vi "Waveform and Laser Controls V4.vi"() -> ()   [LabVIEW 2014]
uses:
  Waveform Scan Parameters.ctl
  <vilib>/Platform/TimedLoop/XDataNode/timing_clust.ctl
  <vilib>/Platform/TimedLoop/XDataNode/nitl_modes.ctl
  <vilib>/Platform/TimedLoop/XDataNode/wakeup.ctl
  <vilib>/rvi/Emulation/niFpgaGetClockAttributes.vi
  <vilib>/rvi/Emulation/niFpgaSctlEmulationGetInTimedLoop.vi
  <vilib>/rvi/Emulation/niFpgaEmulationReportErrorSimple.vi
  <vilib>/rvi/Emulation/niFpgaProcessEmulError.vi
  <vilib>/rvi/eio/common/nirviEmuTemplateMethod_errors.vi
  <vilib>/rvi/Emulation/niFpgaCriticalErrorInLSC.vi
  <vilib>/rvi/Memory/Memory_Emulation/nirvimemoryFastEmulation.vi
  <vilib>/rvi/Memory/Memory_Emulation/nirvimemoryEmulation.vi
  <vilib>/rvi/Emulation/niFpgaEmulationIsFPGAContextNoSignature.vi
  <vilib>/rvi/DataTransferAndStorage/Container/Common/niFpgaContainerGetUniqueNameForEmu.vi
  <vilib>/rvi/errors/nirviReportUnexpectedCaseInternalError (U32).vi
  <vilib>/eio/EIONode/EIONode.xnode
  <vilib>/rvi/DataTransferAndStorage/Container/XNode/niFpgaContainer.xnode
  <vilib>/Platform/TimedLoop/XDataNode/XDataNode.xnode
  <vilib>/Platform/TimedLoop/XDataNode/XDNodeRunTimeDep.lvlib
panel:
  in  "775 AOM (I16)":i16=16500
  in  "590 Analog Voltage (I16)":i16
  out "Laser Blank Trigger":bool
  in  "Laser On Time (Ticks)":u8=8
  in  "Sequences":u8=4
  in  "Laser Delay (Ticks)":u8
  in  "Laser States":u32
  in  "Blanking Off/Manual":bool
  in  "Z Piezo Axis":i16
  in  "Y Piezo Axis":i16
  in  "X Piezo Axis":i16
  out "End Linear Ramp":bool
  in  "End of Linear Ramp":u32
  in  "Z Stack Start Position (I16)":i16
  in  "Frames Per Z Step":u8
  in  "Number of Z Steps":u8
  in  "Z Step Size (I16)":i16
  in  "Stop Sync Signal":bool
  in  "Accums Per Line":u32[](array[numeric])=[0, 0, 0, 0]
  in  "Number of Lines":u32
  out "Frame Trigger":bool
  in  "Reset Position Error":bool
  in  "Galvo 1 Position (I16)":i16
  in  "Galvo 2 Position (I16)":i16
  in  "WF 3 Data Loaded":bool
  in  "WF 2 Data Loaded":bool
  in  "Waveform Scan Parameters":T1={"Scanning Mode"=0, "Fast Axis WF Length (Elements)"=0, "Fast Axis Sample Period (Ticks)"=40, "Slow Axis 1 WF Length (Elements)"=0, "Slow Axis 1 Sample Period (Ticks)"=40, "Slow Axis 1 Delay (25 ns) Steps"=40, "Slow Axis 2 WFLength (Elements)"=0, "Slow Axis 2 Sample Period (Ticks)"=40, "Slow Axis 2 Delay (25 ns) Steps"=40}
  in  "Resonant Mirror":T2
  in  "Galvo Mirror 2":T3
  in  "Galvo Mirror 1":T3
  in  "Start Waveforms":bool
  in  "Unused Axis Offset":i16
  in  "Slow Axis 2 Waveform Element":i16
  in  "Fast Axis Waveform Element":i16
  in  "Slow Axis 1 Waveform Element":i16
  in  "WF 1 Data Loaded":bool
  # "V2 - Adding in a line clock\nV3 - Cluster Scan Parameters"
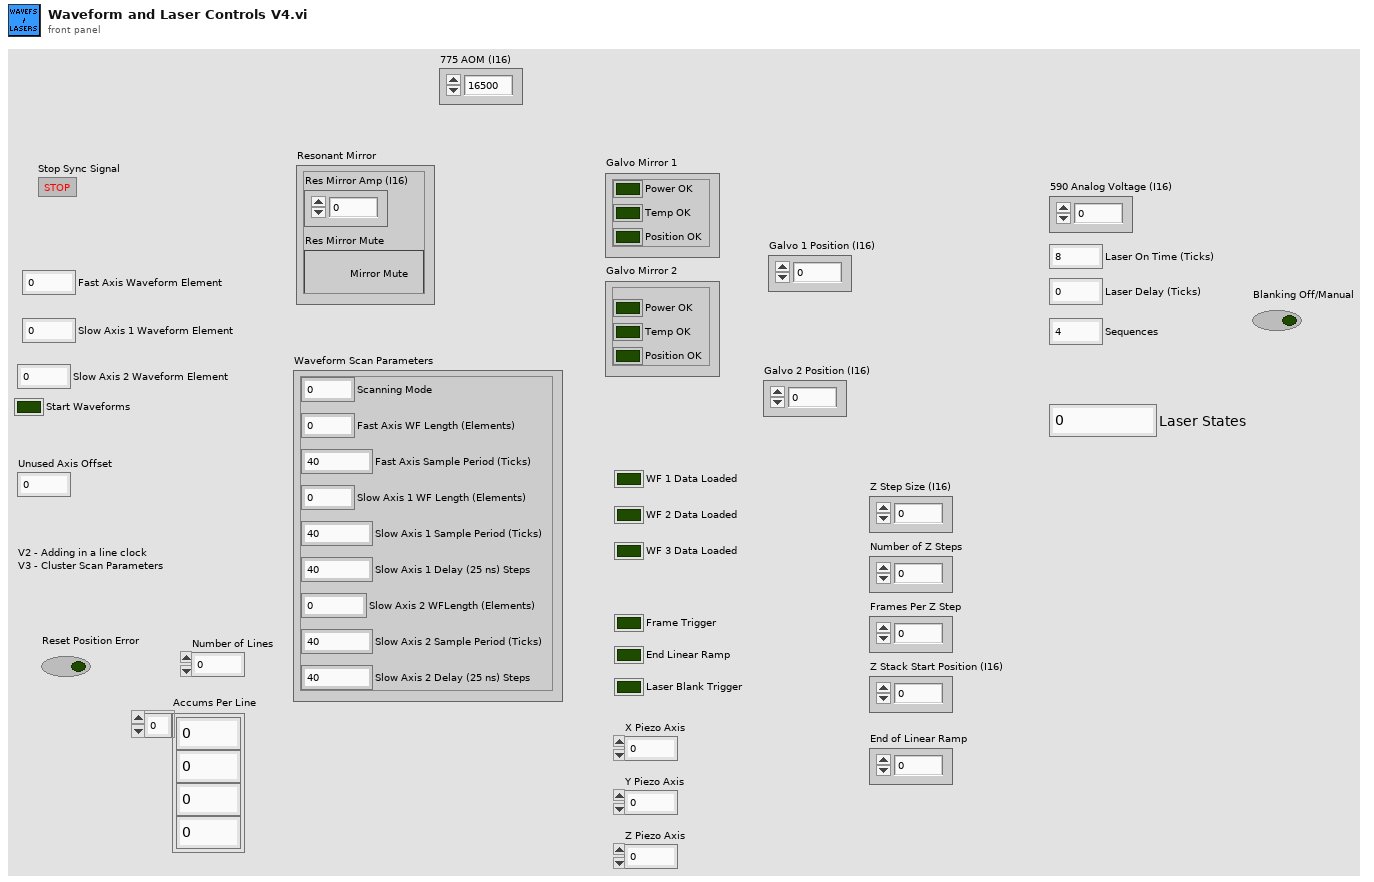
[diagram p1: front panel]
types:
  T1 = typedef "Waveform Scan Parameters.ctl" = cluster{"Scanning Mode":u8, "Fast Axis WF Length (Elements)":i32, "Fast Axis Sample Period (Ticks)":u32, "Slow Axis 1 WF Length (Elements)":i32, "Slow Axis 1 Sample Period (Ticks)":u32, "Slow Axis 1 Delay (25 ns) Steps":i32, "Slow Axis 2 WFLength (Elements)":i32, "Slow Axis 2 Sample Period (Ticks)":u32, "Slow Axis 2 Delay (25 ns) Steps":i32}
  T2 = cluster{"Res Mirror Amp (I16)":i16, "Res Mirror Mute":bool}
  T3 = cluster{"Power OK":bool, "Temp OK":bool, "Position OK":bool}
  T4 = typedef "XDNodeRunTimeDep.lvlib/timing_clust.ctl" = cluster{"Expected End [f-1]":u64, "Actual End [f-1]":u64, "Finished Late? [f-1]":bool, "Expected End [i-1]":u64, "Actual End [i-1]":u64, "Finished Late? [i-1]":bool, "Expected Start [i]":u64, "Actual Start [i]":u64, "Expected Start [f]":u64, "Actual Start [f]":u64, "Source Name":string, "Structure Name":string, "Period":i64, "Deadline":i64, "Offset":i64, "Start":i64, "Priority":i32, "Timeout":i32, "Mode":T5, "Wakeup Reason":T6, "Error":errorcluster, "Source Type":string, "Secondary Source Type":string, "Global End Time":u64, "Global Start Time":u64, "Frame Duration":u64, "Iteration Duration":u64, "Assigned CPU":i32, "I/O Scan Engine Mode":u32}
  T5 = typedef "XDNodeRunTimeDep.lvlib/nitl_modes.ctl" = enum32{"No Change", "Process missed periods, maintain original phase", "Discard missed periods, maintain original phase", "Process missed periods, ignore original phase", "Discard missed periods, ignore original phase"}
  T6 = typedef "XDNodeRunTimeDep.lvlib/wakeup.ctl" = enum32{"Normal", "Aborted", "Asynchronous wakeup", "Timing source error", "Timed loop error", "Timeout"}
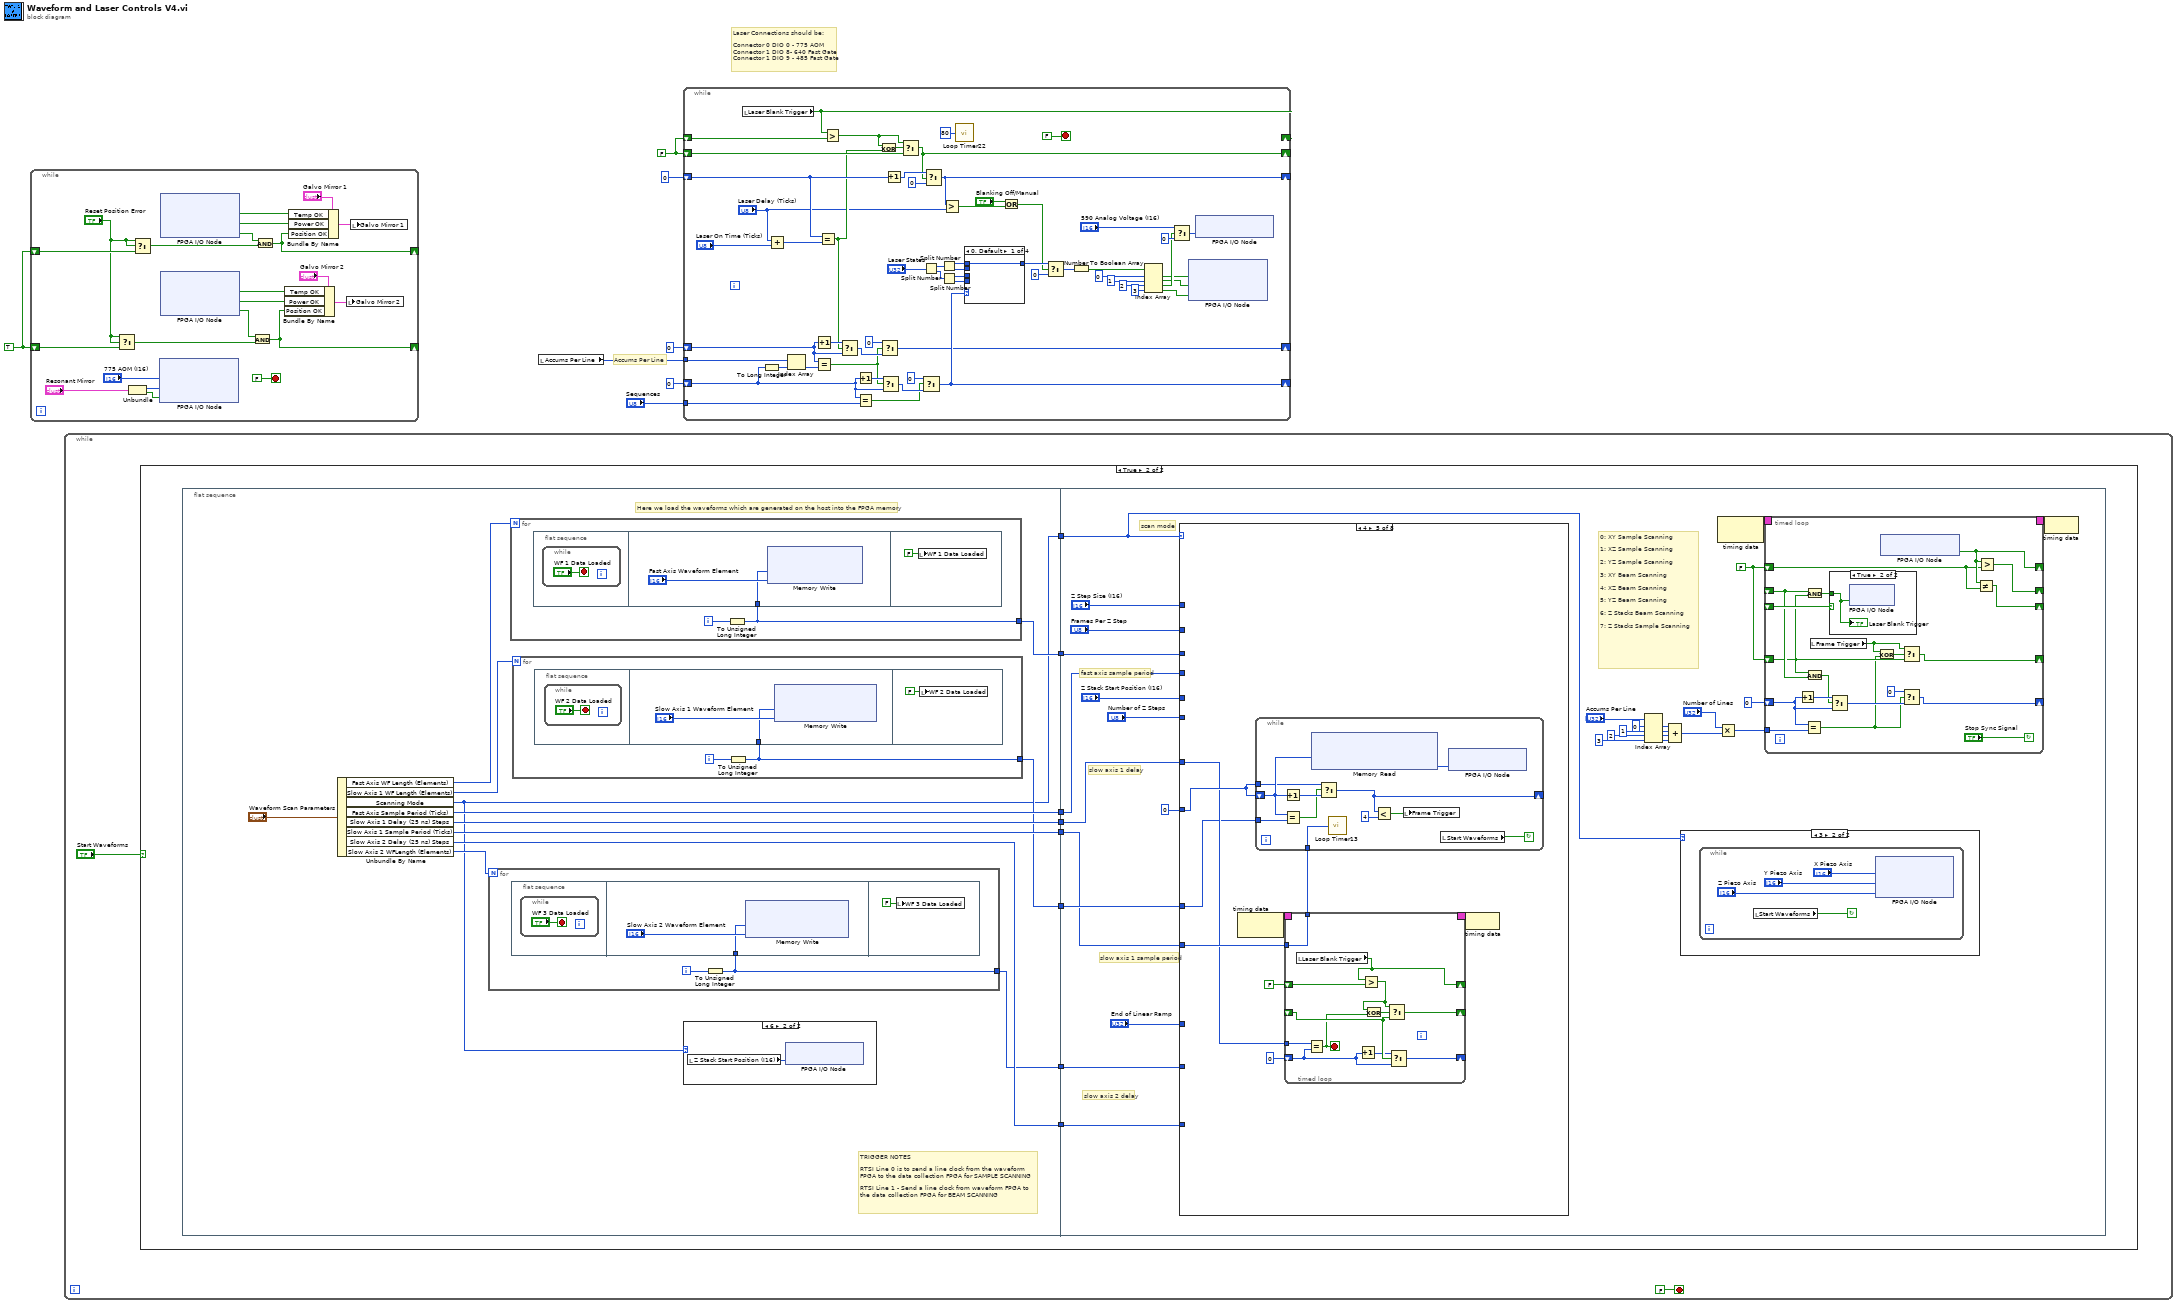
[diagram p0: block diagram]
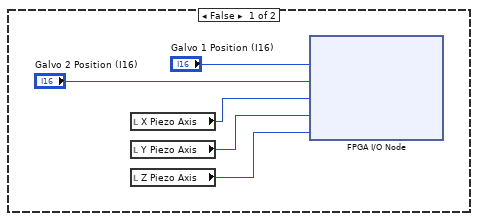
[diagram p5: hidden frame]
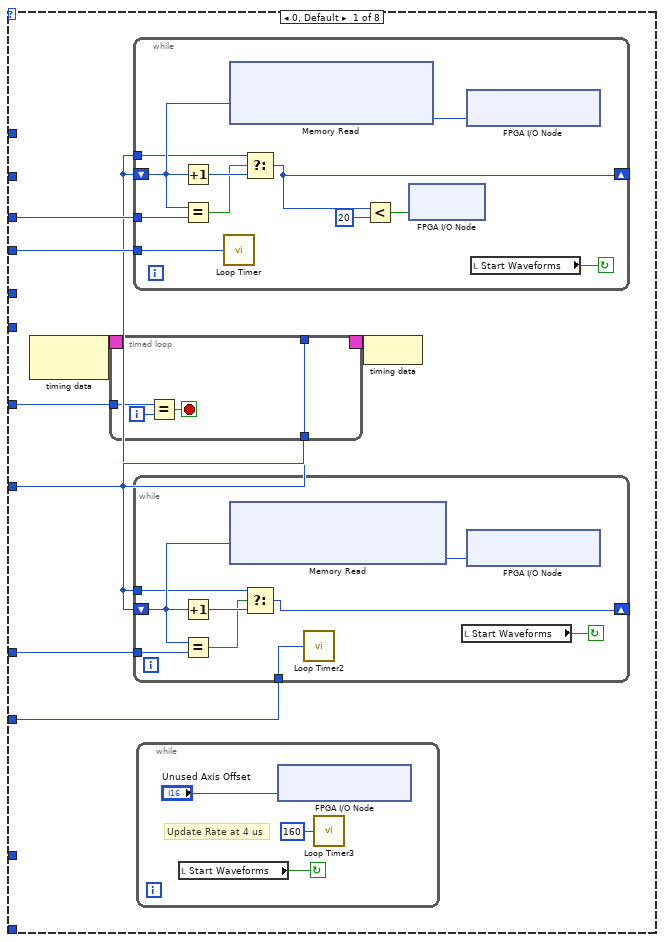
[diagram p9: hidden frame]
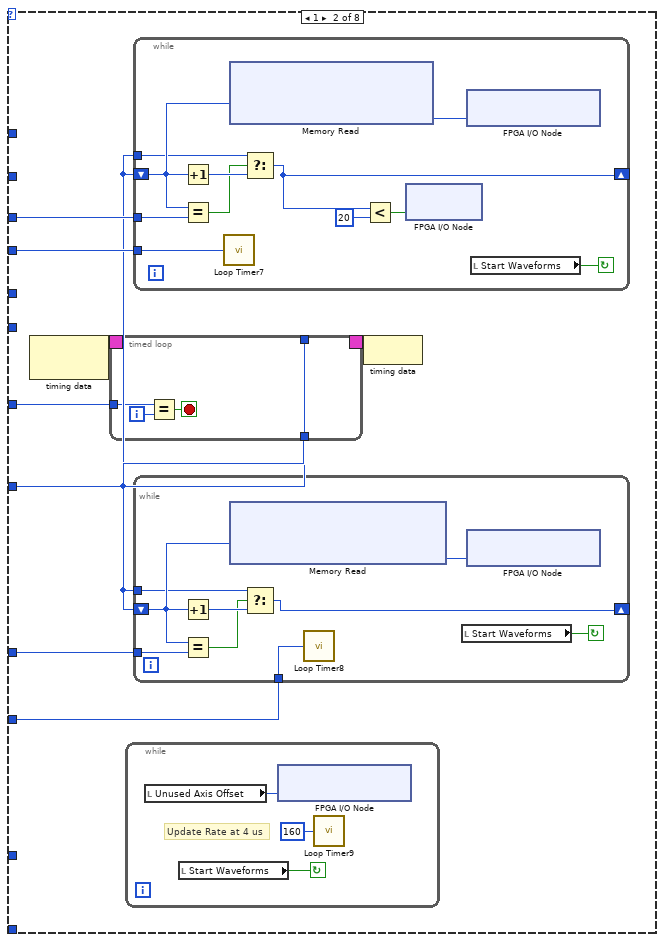
[diagram p10: hidden frame]
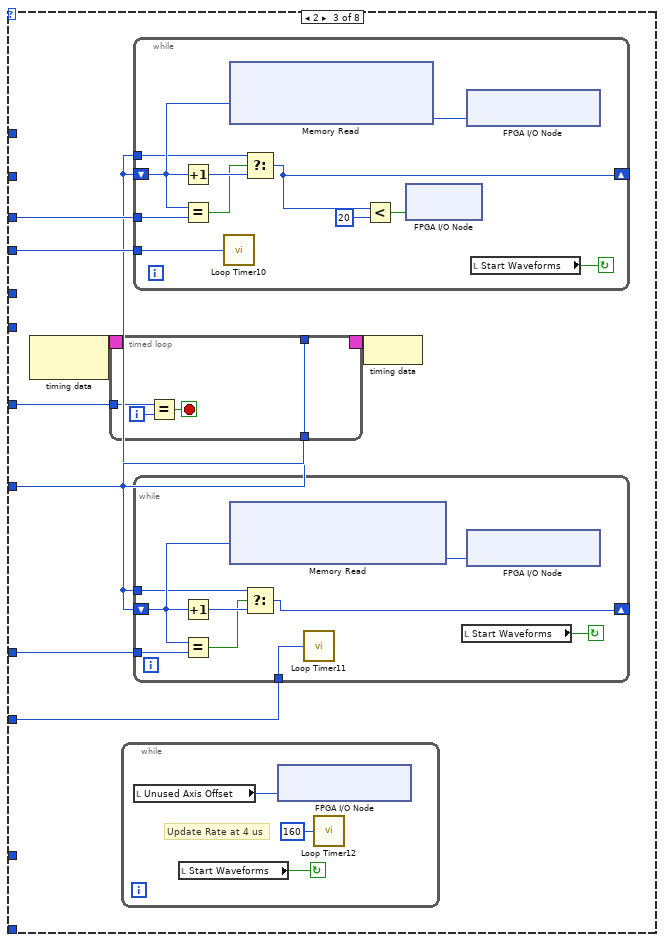
[diagram p11: hidden frame]
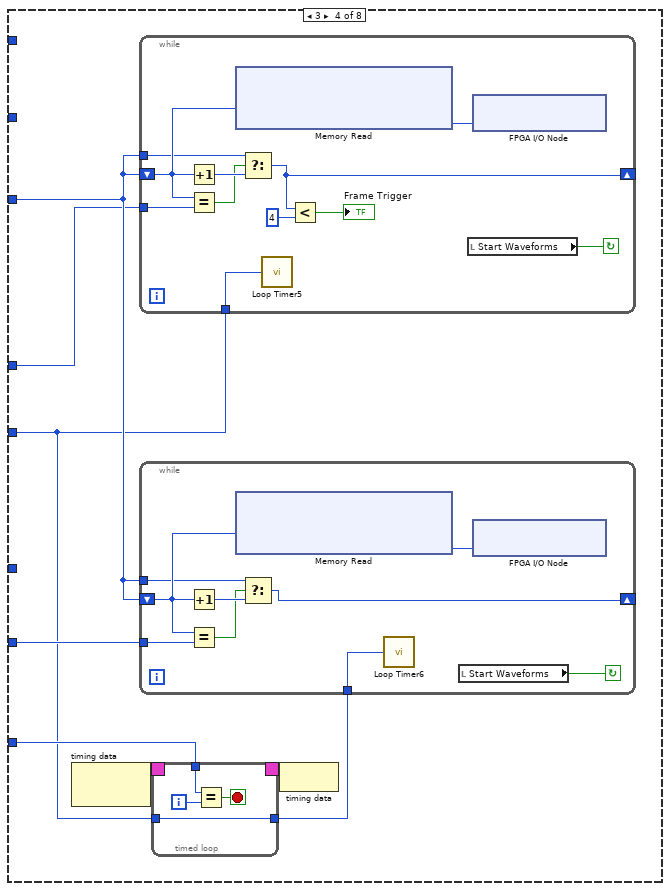
[diagram p12: hidden frame]
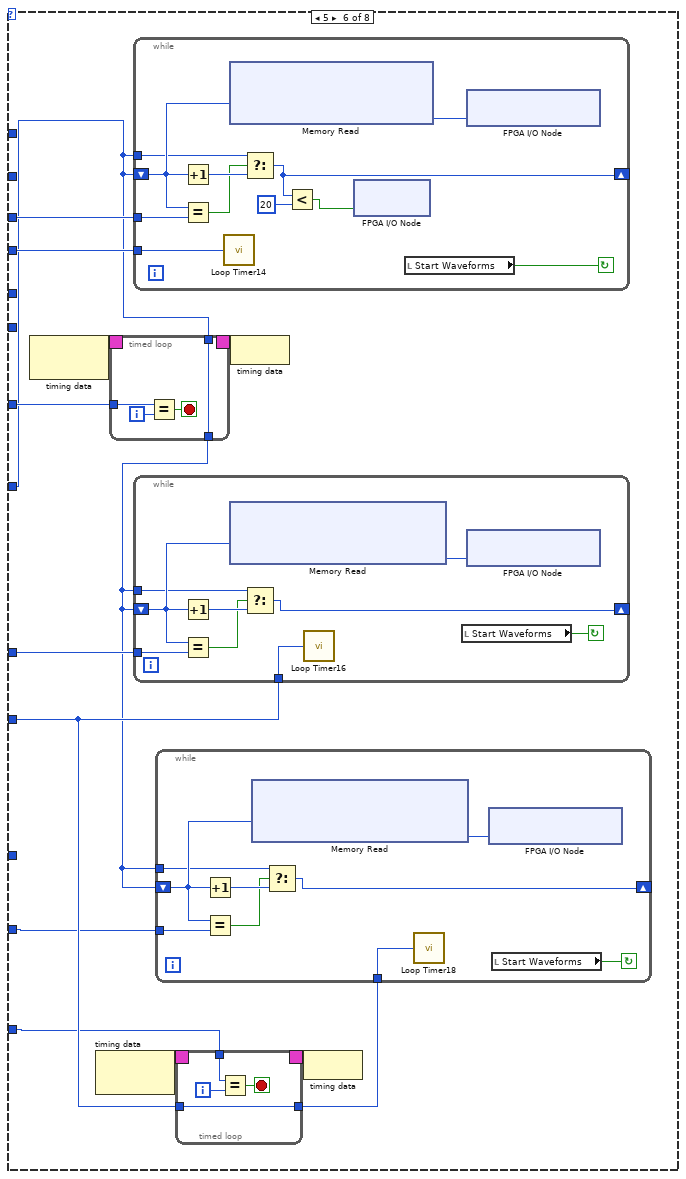
[diagram p13: hidden frame]
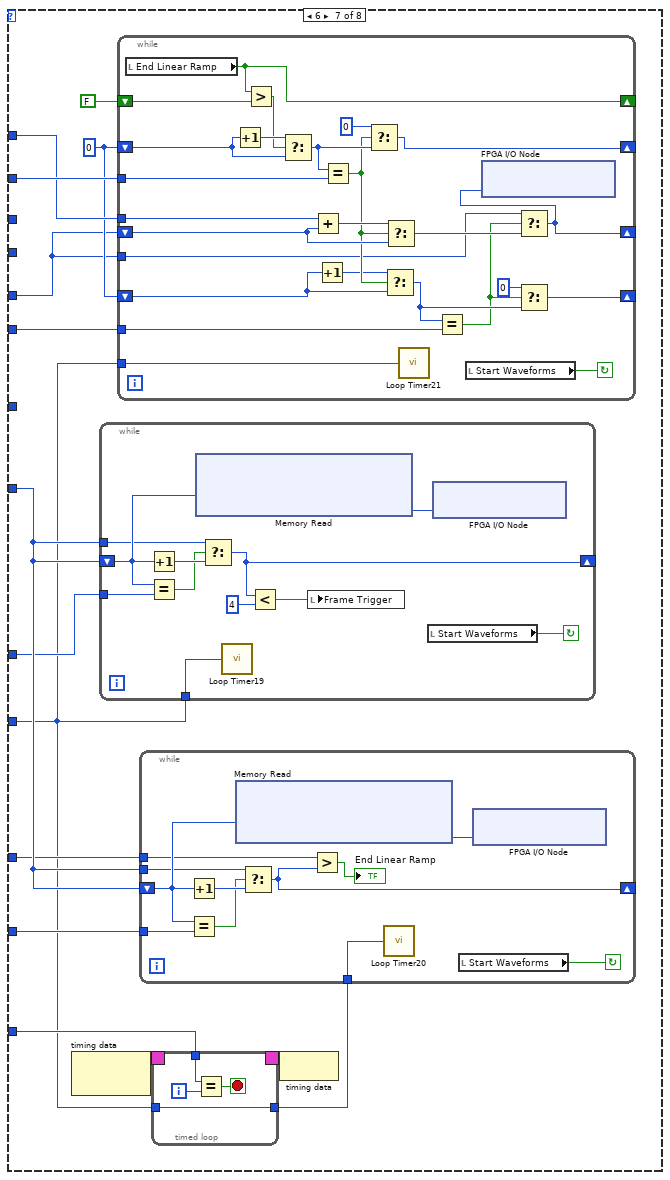
[diagram p14: hidden frame]
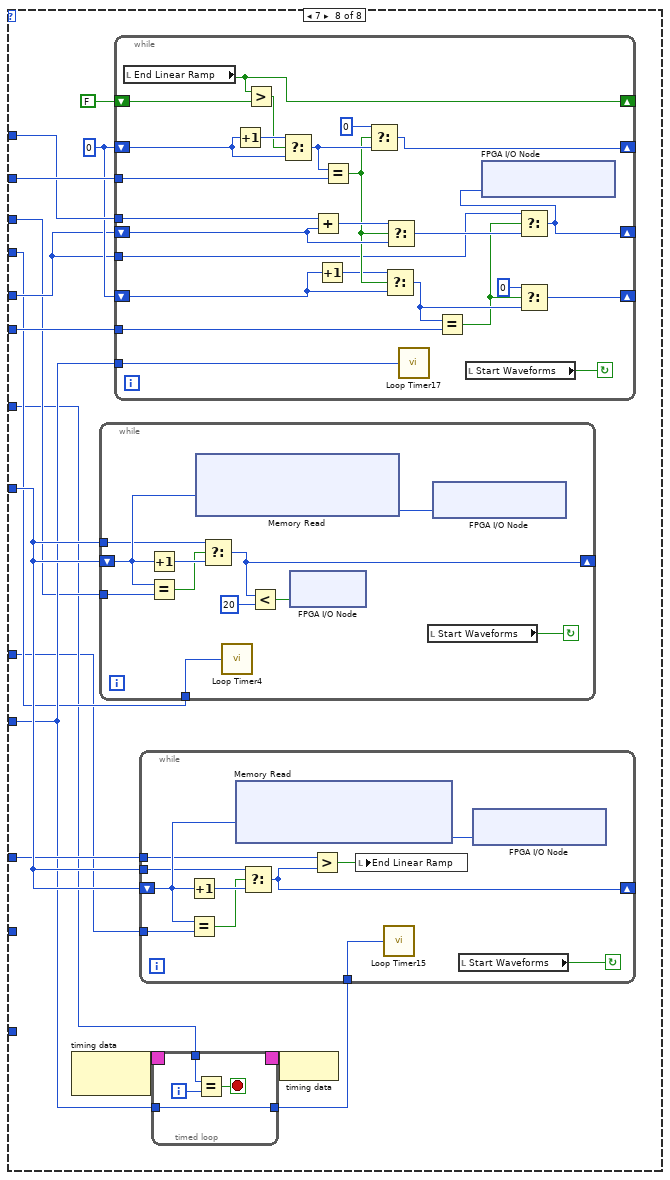
[diagram p15: hidden frame]
diagram:
  w2 = FALSE
  w7 = TRUE
  # "Laser Connections should be:\n\nConnector 0 DIO 0 - 775 AOM\nConnector 1 DIO 8- 640 Fast Gate\nConnector 1 DIO 9 - 485 Fast Gate"
  # "Accums Per Line"
  n1 = while {
    shift-right: [w14] -> _
    shift-left: w7 -> [w16]
    shift-right: [w10] -> _
    shift-left: w7 -> [w12]
    stop <- FALSE stop-if-true
    n2 = Select(t="Reset Position Error", s="Reset Position Error", f=w16) -> (s? t:f=w15:bool)
    n3 = Unbundle("Resonant Mirror") -> ("Res Mirror Amp (I16)"=w27:i16, "Res Mirror Mute"=w26:bool)
    n4 = Select(t="Reset Position Error", s="Reset Position Error", f=w12) -> (s? t:f=w11:bool)
    n5 = xnode "FPGA I/O Node"("Connector0/AO4"="775 AOM (I16)", "Connector0/AO7"=w27, "Connector0/DIO7"=w26) -> ()  [unwired: 4 in, 4 out]
    n6 = xnode "FPGA I/O Node"() -> ("Connector0/DIO1"=w25:bool, "Connector0/DIO2"=w24:bool, "Connector0/DIO3"=w13:bool)  [unwired: 4 in, 4 out]
    n7 = xnode "FPGA I/O Node"() -> ("Connector0/DIO4"=w18:bool, "Connector0/DIO5"=w19:bool, "Connector0/DIO6"=w17:bool)  [unwired: 4 in, 4 out]
    n8 = And(x=w17, y=w15) -> (x .and. y?=w14:bool)
    n9 = And(x=w13, y=w11) -> (x .and. y?=w10:bool)
    n10 = Bundle By Name(cluster="Galvo Mirror 2", "Temp OK"=w18, "Power OK"=w19, "Position OK"=w14) -> (w21:T3)
    n11 = Bundle By Name(cluster="Galvo Mirror 1", "Temp OK"=w25, "Power OK"=w24, "Position OK"=w10) -> (w23:T3)
    n12 = local write "Galvo Mirror 2"(w21) -> ()
    n13 = local write "Galvo Mirror 1"(w23) -> ()
  }
  n14 = while {
    stop <- FALSE stop-if-true
    n15 = case shown="True" "Start Waveforms" {
      frame False {
        n16 = local read "X Piezo Axis"() -> (w34:i16)
        n17 = local read "Y Piezo Axis"() -> (w33:i16)
        n18 = local read "Z Piezo Axis"() -> (w32:i16)
        n19 = xnode "FPGA I/O Node"("Connector0/AO5"="Galvo 1 Position (I16)", "Connector0/AO6"="Galvo 2 Position (I16)", "Connector0/AO1"=w34, "Connector0/AO2"=w33, "Connector0/AO3"=w32) -> ()  [unwired: 5 in, 5 out]
      }
      frame True {
        n20 = flat-sequence {
          tunnel: [w56] -> w44
          tunnel: [w46] -> w43
          tunnel: [w47] -> w42
          tunnel: [w45] -> w41
          tunnel: [w54] -> w40
          tunnel: [w53] -> w39
          tunnel: [w52] -> w38
          tunnel: [w51] -> w37
          tunnel: w44 -> [w105]
          tunnel: w43 -> [w104]
          tunnel: w42 -> [w102]
          tunnel: w41 -> [w76]
          tunnel: w40 -> [w101]
          tunnel: w39 -> [w100]
          tunnel: w38 -> [w99]
          tunnel: w37 -> [w98]
          frame #0 {
            # "TRIGGER NOTES\n\nRTSI Line 0 is to send a line clock from the waveform\nFPGA to the data collection FPGA for SAMPLE SCANNING\n\nRTSI Line 1 - Send a line clock from waveform FPGA to\nthe data collection FPGA for BEAM SCANNING"
            # "Here we load the waveforms which are generated on the host into the FPGA memory"
            n21 = Unbundle By Name("Waveform Scan Parameters") -> ("Fast Axis WF Length (Elements)"=w50:i32, "Slow Axis 1 WF Length (Elements)"=w49:i32, "Scanning Mode"=w45:u8, "Fast Axis Sample Period (Ticks)"=w54:u32, "Slow Axis 1 Delay (25 ns) Steps"=w53:i32, "Slow Axis 1 Sample Period (Ticks)"=w52:u32, "Slow Axis 2 Delay (25 ns) Steps"=w51:i32, "Slow Axis 2 WFLength (Elements)"=w48:i32)
            n22 = for {
              N: w48 -> [_]
              tunnel: [w58] -> w46
              i -> [w59]
              n23 = flat-sequence {
                tunnel: w58 -> [w61]
                frame #0 {
                  n24 = while {
                    stop <- "WF 3 Data Loaded" stop-if-true
                  }
                }
                frame #1 {
                  n25 = xnode ("Memory Write")("Address"=w61, "Data"="Slow Axis 2 Waveform Element") -> ()  [unwired: 1 in, 1 out]
                }
                frame #2 {
                  n26 = local write "WF 3 Data Loaded"(FALSE ("Host Data Loaded")) -> ()
                }
              }
              n27 = To Unsigned Long Integer(number=w59) -> (unsigned 32bit integer=w58:u32)
            }
            n28 = for {
              N: w50 -> [_]
              tunnel: [w70] -> w56
              i -> [w71]
              n29 = flat-sequence {
                tunnel: w70 -> [w73]
                frame #0 {
                  n30 = while {
                    stop <- "WF 1 Data Loaded" stop-if-true
                  }
                }
                frame #1 {
                  n31 = xnode ("Memory Write")("Address"=w73, "Data"="Fast Axis Waveform Element") -> ()  [unwired: 1 in, 1 out]
                }
                frame #2 {
                  n32 = local write "WF 1 Data Loaded"(FALSE ("Host Data Loaded")) -> ()
                }
              }
              n33 = To Unsigned Long Integer(number=w71) -> (unsigned 32bit integer=w70:u32)
            }
            n34 = for {
              N: w49 -> [_]
              tunnel: [w64] -> w47
              i -> [w65]
              n35 = flat-sequence {
                tunnel: w64 -> [w67]
                frame #0 {
                  n36 = while {
                    stop <- "WF 2 Data Loaded" stop-if-true
                  }
                }
                frame #1 {
                  n37 = xnode ("Memory Write")("Address"=w67, "Data"="Slow Axis 1 Waveform Element") -> ()  [unwired: 1 in, 1 out]
                }
                frame #2 {
                  n38 = local write "WF 2 Data Loaded"(FALSE ("Host Data Loaded")) -> ()
                }
              }
              n39 = To Unsigned Long Integer(number=w65) -> (unsigned 32bit integer=w64:u32)
            }
            n40 = case shown="6" w45 {
              frame 0, Default {
              }
              frame 6 {
                n41 = local read "Z Stack Start Position (I16)"() -> (w57:i16)
                n42 = xnode "FPGA I/O Node"("Connector0/AO3"=w57) -> ()  [unwired: 1 in, 1 out]
              }
            }
          }
          frame #1 {
            w83 = FALSE
            # "slow axis 2 delay"
            # "slow axis 1 sample period"
            # "slow axis 1 delay"
            # "fast axis sample period"
            # "scan mode"
            # "0: XY Sample Scanning\n\n1: XZ Sample Scanning\n\n2: YZ Sample Scanning\n\n3: XY Beam Scanning\n\n4: XZ Beam Scanning\n\n5: YZ Beam Scanning\n\n6: Z Stacks Beam Scanning\n\n7: Z Stacks Sample Scanning"
            n43 = case shown="4" w76 {
              tunnel: w105 -> [w141 w181 w221 _ _ w340 _ w458]
              tunnel: w101 -> [w140 w180 w220 _ _ w339 _ w459]
              tunnel: w104 -> [_ _ _ w262 _ w334 w400 _]
              tunnel: u32 0 -> [w135 w175 w215 w261 w299 w336 w399 w471]
              tunnel: w100 -> [w139 w179 w219 _ w297 w338 _ w457]
              tunnel: w98 -> [_ _ _ w260 _ w333 w398 _]
              tunnel: w102 -> [w137 w177 w217 w255 w296 w337 w395 w456]
              tunnel: w99 -> [w136 w176 w216 w256 w298 w335 w386 w460]
              tunnel: "Frames Per Z Step" -> [_ _ _ _ _ _ w393 w467]
              tunnel: "Z Stack Start Position (I16)" -> [_ _ _ _ _ _ w389 w463]
              tunnel: "Z Step Size (I16)" -> [_ _ _ _ _ _ w392 w466]
              tunnel: "Number of Z Steps" -> [_ _ _ _ _ _ w390 w464]
              tunnel: "End of Linear Ramp" -> [_ _ _ _ _ _ w388 w462]
              frame 0, Default {
                n44 = node-c288() -> (w143:T4)  [unwired: 1 in]
                n45 = timed-loop {
                  timing: w143 -> [_]
                  timing-out: [_] -> w142
                  tunnel: w139 -> [w148]
                  tunnel: w135 -> [w147]
                  tunnel: [w147] -> w138
                  i -> [w150]
                  stop <- w149 stop-if-true
                  n46 = Equal?(x=w148, y=w150) -> (x = y?=w149:bool)
                }
                n47 = while {
                  shift-right: [w166] -> _
                  shift-left: w135 -> [w172]
                  tunnel: w141 -> [w173]
                  tunnel: w140 -> [w170]
                  tunnel: w135 -> [w169]
                  stop <- w168 continue-if-true
                  n48 = Increment(x=w172) -> (x+1=w174:u32)
                  n49 = Equal?(x=w172, y=w173) -> (x = y?=w167:bool)
                  n50 = call "Loop Timer"("Count(Ticks)"=w170) -> ()  [unwired: 1 out]
                  n51 = xnode ("Memory Read")("Address"=w172) -> ("Data"=w171:i16)  [unwired: 1 in, 1 out]
                  n52 = Select(t=w169, s=w167, f=w174) -> (s? t:f=w166:u32)
                  n53 = Less?(x=w166, y=u32 20) -> (x < y?=w164:bool)
                  n54 = xnode "FPGA I/O Node"("TRIG0"=w164) -> ()  [unwired: 1 in, 1 out]
                  n55 = xnode "FPGA I/O Node"("Connector0/AO1"=w171) -> ()  [unwired: 1 in, 1 out]
                  n56 = local read "Start Waveforms"() -> (w168:bool)
                }
                n57 = while {
                  shift-right: [w162] -> _
                  shift-left: w138 -> [w159]
                  tunnel: w137 -> [w161]
                  tunnel: w138 -> [w157]
                  tunnel: w136 -> [w156]
                  stop <- w155 continue-if-true
                  n58 = Increment(x=w159) -> (x+1=w163:u32)
                  n59 = Equal?(x=w159, y=w161) -> (x = y?=w160:bool)
                  n60 = xnode ("Memory Read")("Address"=w159) -> ("Data"=w158:i16)  [unwired: 1 in, 1 out]
                  n61 = Select(t=w157, s=w160, f=w163) -> (s? t:f=w162:u32)
                  n62 = call "Loop Timer2"("Count(Ticks)"=w156) -> ()  [unwired: 1 out]
                  n63 = local read "Start Waveforms"() -> (w155:bool)
                  n64 = xnode "FPGA I/O Node"("Connector0/AO2"=w158) -> ()  [unwired: 1 in, 1 out]
                }
                n65 = while {
                  stop <- w144 continue-if-true
                  # "Update Rate at 4 us"
                  n66 = local read "Start Waveforms"() -> (w144:bool)
                  n67 = xnode "FPGA I/O Node"("Connector0/AO3"="Unused Axis Offset") -> ()  [unwired: 1 in, 1 out]
                  n68 = call "Loop Timer3"("Count(Ticks)"=u32 160) -> ()  [unwired: 1 out]
                }
                n69 = node-c288(w142) -> ()
              }
              frame 1 {
                n70 = node-c288() -> (w183:T4)  [unwired: 1 in]
                n71 = timed-loop {
                  timing: w183 -> [_]
                  timing-out: [_] -> w182
                  tunnel: w179 -> [w188]
                  tunnel: w175 -> [w187]
                  tunnel: [w187] -> w178
                  i -> [w190]
                  stop <- w189 stop-if-true
                  n72 = Equal?(x=w188, y=w190) -> (x = y?=w189:bool)
                }
                n73 = while {
                  stop <- w185 continue-if-true
                  # "Update Rate at 4 us"
                  n74 = local read "Unused Axis Offset"() -> (w184:i16)
                  n75 = local read "Start Waveforms"() -> (w185:bool)
                  n76 = xnode "FPGA I/O Node"("Connector0/AO2"=w184) -> ()  [unwired: 1 in, 1 out]
                  n77 = call "Loop Timer9"("Count(Ticks)"=u32 160) -> ()  [unwired: 1 out]
                }
                n78 = while {
                  shift-right: [w206] -> _
                  shift-left: w175 -> [w212]
                  tunnel: w181 -> [w213]
                  tunnel: w180 -> [w210]
                  tunnel: w175 -> [w209]
                  stop <- w208 continue-if-true
                  n79 = Increment(x=w212) -> (x+1=w214:u32)
                  n80 = Equal?(x=w212, y=w213) -> (x = y?=w207:bool)
                  n81 = call "Loop Timer7"("Count(Ticks)"=w210) -> ()  [unwired: 1 out]
                  n82 = xnode ("Memory Read")("Address"=w212) -> ("Data"=w211:i16)  [unwired: 1 in, 1 out]
                  n83 = Select(t=w209, s=w207, f=w214) -> (s? t:f=w206:u32)
                  n84 = Less?(x=w206, y=u32 20) -> (x < y?=w204:bool)
                  n85 = xnode "FPGA I/O Node"("TRIG0"=w204) -> ()  [unwired: 1 in, 1 out]
                  n86 = xnode "FPGA I/O Node"("Connector0/AO1"=w211) -> ()  [unwired: 1 in, 1 out]
                  n87 = local read "Start Waveforms"() -> (w208:bool)
                }
                n88 = while {
                  shift-right: [w202] -> _
                  shift-left: w178 -> [w199]
                  tunnel: w177 -> [w201]
                  tunnel: w178 -> [w197]
                  tunnel: w176 -> [w196]
                  stop <- w195 continue-if-true
                  n89 = Increment(x=w199) -> (x+1=w203:u32)
                  n90 = Equal?(x=w199, y=w201) -> (x = y?=w200:bool)
                  n91 = xnode ("Memory Read")("Address"=w199) -> ("Data"=w198:i16)  [unwired: 1 in, 1 out]
                  n92 = Select(t=w197, s=w200, f=w203) -> (s? t:f=w202:u32)
                  n93 = call "Loop Timer8"("Count(Ticks)"=w196) -> ()  [unwired: 1 out]
                  n94 = local read "Start Waveforms"() -> (w195:bool)
                  n95 = xnode "FPGA I/O Node"("Connector0/AO3"=w198) -> ()  [unwired: 1 in, 1 out]
                }
                n96 = node-c288(w182) -> ()
              }
              frame 2 {
                n97 = node-c288() -> (w223:T4)  [unwired: 1 in]
                n98 = timed-loop {
                  timing: w223 -> [_]
                  timing-out: [_] -> w222
                  tunnel: w219 -> [w228]
                  tunnel: w215 -> [w227]
                  tunnel: [w227] -> w218
                  i -> [w230]
                  stop <- w229 stop-if-true
                  n99 = Equal?(x=w228, y=w230) -> (x = y?=w229:bool)
                }
                n100 = while {
                  stop <- w225 continue-if-true
                  # "Update Rate at 4 us"
                  n101 = local read "Unused Axis Offset"() -> (w224:i16)
                  n102 = local read "Start Waveforms"() -> (w225:bool)
                  n103 = xnode "FPGA I/O Node"("Connector0/AO1"=w224) -> ()  [unwired: 1 in, 1 out]
                  n104 = call "Loop Timer12"("Count(Ticks)"=u32 160) -> ()  [unwired: 1 out]
                }
                n105 = while {
                  shift-right: [w246] -> _
                  shift-left: w215 -> [w252]
                  tunnel: w221 -> [w253]
                  tunnel: w220 -> [w250]
                  tunnel: w215 -> [w249]
                  stop <- w248 continue-if-true
                  n106 = Increment(x=w252) -> (x+1=w254:u32)
                  n107 = Equal?(x=w252, y=w253) -> (x = y?=w247:bool)
                  n108 = call "Loop Timer10"("Count(Ticks)"=w250) -> ()  [unwired: 1 out]
                  n109 = xnode ("Memory Read")("Address"=w252) -> ("Data"=w251:i16)  [unwired: 1 in, 1 out]
                  n110 = Select(t=w249, s=w247, f=w254) -> (s? t:f=w246:u32)
                  n111 = Less?(x=w246, y=u32 20) -> (x < y?=w244:bool)
                  n112 = xnode "FPGA I/O Node"("TRIG0"=w244) -> ()  [unwired: 1 in, 1 out]
                  n113 = xnode "FPGA I/O Node"("Connector0/AO2"=w251) -> ()  [unwired: 1 in, 1 out]
                  n114 = local read "Start Waveforms"() -> (w248:bool)
                }
                n115 = while {
                  shift-right: [w242] -> _
                  shift-left: w218 -> [w239]
                  tunnel: w217 -> [w241]
                  tunnel: w218 -> [w237]
                  tunnel: w216 -> [w236]
                  stop <- w235 continue-if-true
                  n116 = Increment(x=w239) -> (x+1=w243:u32)
                  n117 = Equal?(x=w239, y=w241) -> (x = y?=w240:bool)
                  n118 = xnode ("Memory Read")("Address"=w239) -> ("Data"=w238:i16)  [unwired: 1 in, 1 out]
                  n119 = Select(t=w237, s=w240, f=w243) -> (s? t:f=w242:u32)
                  n120 = call "Loop Timer11"("Count(Ticks)"=w236) -> ()  [unwired: 1 out]
                  n121 = local read "Start Waveforms"() -> (w235:bool)
                  n122 = xnode "FPGA I/O Node"("Connector0/AO3"=w238) -> ()  [unwired: 1 in, 1 out]
                }
                n123 = node-c288(w222) -> ()
              }
              frame 3 {
                n124 = node-c288() -> (w259:T4)  [unwired: 1 in]
                n125 = while {
                  shift-right: [w282] -> _
                  shift-left: w261 -> [w288]
                  tunnel: w255 -> [w289]
                  tunnel: w256 -> [w286]
                  tunnel: w261 -> [w285]
                  stop <- w284 continue-if-true
                  n126 = Increment(x=w288) -> (x+1=w290:u32)
                  n127 = Equal?(x=w288, y=w289) -> (x = y?=w283:bool)
                  n128 = xnode ("Memory Read")("Address"=w288) -> ("Data"=w287:i16)  [unwired: 1 in, 1 out]
                  n129 = Select(t=w285, s=w283, f=w290) -> (s? t:f=w282:u32)
                  n130 = call "Loop Timer5"("Count(Ticks)"=w286) -> ()  [unwired: 1 out]
                  n131 = Less?(x=w282, y=u32 4) -> (x < y?=→"Frame Trigger":bool)
                  n132 = local read "Start Waveforms"() -> (w284:bool)
                  n133 = xnode "FPGA I/O Node"("Connector0/AO5"=w287) -> ()  [unwired: 1 in, 1 out]
                }
                n134 = timed-loop {
                  timing: w259 -> [_]
                  timing-out: [_] -> w258
                  tunnel: w256 -> [w272]
                  tunnel: [w272] -> w257
                  tunnel: w260 -> [w273]
                  i -> [w275]
                  stop <- w274 stop-if-true
                  n135 = Equal?(x=w273, y=w275) -> (x = y?=w274:bool)
                }
                n136 = while {
                  shift-right: [w270] -> _
                  shift-left: w261 -> [w268]
                  tunnel: w262 -> [w269]
                  tunnel: w257 -> [w266]
                  tunnel: w261 -> [w265]
                  stop <- w264 continue-if-true
                  n137 = Increment(x=w268) -> (x+1=w271:u32)
                  n138 = Equal?(x=w268, y=w269) -> (x = y?=w263:bool)
                  n139 = xnode ("Memory Read")("Address"=w268) -> ("Data"=w267:i16)  [unwired: 1 in, 1 out]
                  n140 = Select(t=w265, s=w263, f=w271) -> (s? t:f=w270:u32)
                  n141 = call "Loop Timer6"("Count(Ticks)"=w266) -> ()  [unwired: 1 out]
                  n142 = local read "Start Waveforms"() -> (w264:bool)
                  n143 = xnode "FPGA I/O Node"("Connector0/AO6"=w267) -> ()  [unwired: 1 in, 1 out]
                }
                n144 = node-c288(w258) -> ()
              }
              frame 4 {
                n145 = node-c288() -> (w295:T4)  [unwired: 1 in]
                n146 = timed-loop {
                  timing: w295 -> [_]
                  timing-out: [_] -> w294
                  tunnel: w298 -> [w302]
                  shift-right: [w300] -> _
                  shift-left: FALSE -> [w311]
                  shift-right: [w308] -> _
                  shift-left: _ -> [w307]
                  shift-right: [w305] -> _
                  shift-left: 0 -> [w303]
                  tunnel: w297 -> [w304]
                  tunnel: [w302] -> w291
                  stop <- w301 stop-if-true
                  n147 = local read "Laser Blank Trigger"() -> (w300:bool)
                  n148 = Equal?(x=w304, y=w303) -> (x = y?=w301:bool)
                  n149 = Increment(x=w303) -> (x+1=w306:i32)
                  n150 = Greater?(x=w300, y=w311) -> (0:w309:bool)
                  n151 = Exclusive Or(1:w301, 2:w309) -> (0:w310:bool)
                  n152 = Select(t=w309, s=w310, f=w307) -> (s? t:f=w308:bool)
                  n153 = Select(t=w306, s=w307, f=w303) -> (s? t:f=w305:i32)
                }
                n154 = while {
                  shift-right: [w317] -> _
                  shift-left: w299 -> [w323]
                  tunnel: w296 -> [w325]
                  tunnel: w291 -> [w321]
                  tunnel: w299 -> [w320]
                  stop <- w319 continue-if-true
                  n155 = Increment(x=w323) -> (x+1=w326:u32)
                  n156 = Equal?(x=w323, y=w325) -> (x = y?=w324:bool)
                  n157 = xnode ("Memory Read")("Address"=w323) -> ("Data"=w322:i16)  [unwired: 1 in, 1 out]
                  n158 = Select(t=w320, s=w324, f=w326) -> (s? t:f=w317:u32)
                  n159 = call "Loop Timer13"("Count(Ticks)"=w321) -> ()  [unwired: 1 out]
                  n160 = Less?(x=w317, y=u32 4) -> (x < y?=w316:bool)
                  n161 = local write "Frame Trigger"(w316) -> ()
                  n162 = local read "Start Waveforms"() -> (w319:bool)
                  n163 = xnode "FPGA I/O Node"("Connector0/AO3"=w322) -> ()  [unwired: 1 in, 1 out]
                }
                n164 = node-c288(w294) -> ()
              }
              frame 5 {
                n165 = node-c288() -> (w332:T4)  [unwired: 1 in]
                n166 = node-c288() -> (w330:T4)  [unwired: 1 in]
                n167 = timed-loop {
                  timing: w332 -> [_]
                  timing-out: [_] -> w331
                  tunnel: w338 -> [w359]
                  tunnel: w336 -> [w358]
                  tunnel: [w358] -> w327
                  i -> [w361]
                  stop <- w360 stop-if-true
                  n168 = Equal?(x=w359, y=w361) -> (x = y?=w360:bool)
                }
                n169 = while {
                  shift-right: [w378] -> _
                  shift-left: w336 -> [w383]
                  tunnel: w340 -> [w384]
                  tunnel: w339 -> [w381]
                  tunnel: w336 -> [w380]
                  stop <- w376 continue-if-true
                  n170 = Increment(x=w383) -> (x+1=w385:u32)
                  n171 = Equal?(x=w383, y=w384) -> (x = y?=w379:bool)
                  n172 = call "Loop Timer14"("Count(Ticks)"=w381) -> ()  [unwired: 1 out]
                  n173 = xnode ("Memory Read")("Address"=w383) -> ("Data"=w382:i16)  [unwired: 1 in, 1 out]
                  n174 = Select(t=w380, s=w379, f=w385) -> (s? t:f=w378:u32)
                  n175 = Less?(x=w378, y=u32 20) -> (x < y?=w375:bool)
                  n176 = xnode "FPGA I/O Node"("TRIG0"=w375) -> ()  [unwired: 1 in, 1 out]
                  n177 = local read "Start Waveforms"() -> (w376:bool)
                  n178 = xnode "FPGA I/O Node"("Connector0/AO5"=w382) -> ()  [unwired: 1 in, 1 out]
                }
                n179 = while {
                  shift-right: [w373] -> _
                  shift-left: w327 -> [w370]
                  tunnel: w337 -> [w372]
                  tunnel: w327 -> [w368]
                  tunnel: w335 -> [w367]
                  stop <- w366 continue-if-true
                  n180 = Increment(x=w370) -> (x+1=w374:u32)
                  n181 = Equal?(x=w370, y=w372) -> (x = y?=w371:bool)
                  n182 = xnode ("Memory Read")("Address"=w370) -> ("Data"=w369:i16)  [unwired: 1 in, 1 out]
                  n183 = Select(t=w368, s=w371, f=w374) -> (s? t:f=w373:u32)
                  n184 = call "Loop Timer16"("Count(Ticks)"=w367) -> ()  [unwired: 1 out]
                  n185 = local read "Start Waveforms"() -> (w366:bool)
                  n186 = xnode "FPGA I/O Node"("Connector0/AO6"=w369) -> ()  [unwired: 1 in, 1 out]
                }
                n187 = timed-loop {
                  timing: w330 -> [_]
                  timing-out: [_] -> w329
                  tunnel: w335 -> [w350]
                  tunnel: [w350] -> w328
                  tunnel: w333 -> [w351]
                  i -> [w353]
                  stop <- w352 stop-if-true
                  n188 = Equal?(x=w351, y=w353) -> (x = y?=w352:bool)
                }
                n189 = while {
                  shift-right: [w348] -> _
                  shift-left: w327 -> [w345]
                  tunnel: w334 -> [w347]
                  tunnel: w328 -> [w343]
                  tunnel: w327 -> [w342]
                  stop <- w341 continue-if-true
                  n190 = Increment(x=w345) -> (x+1=w349:u32)
                  n191 = Equal?(x=w345, y=w347) -> (x = y?=w346:bool)
                  n192 = xnode ("Memory Read")("Address"=w345) -> ("Data"=w344:i16)  [unwired: 1 in, 1 out]
                  n193 = Select(t=w342, s=w346, f=w349) -> (s? t:f=w348:u32)
                  n194 = call "Loop Timer18"("Count(Ticks)"=w343) -> ()  [unwired: 1 out]
                  n195 = xnode "FPGA I/O Node"("Connector0/AO3"=w344) -> ()  [unwired: 1 in, 1 out]
                  n196 = local read "Start Waveforms"() -> (w341:bool)
                }
                n197 = node-c288(w331) -> ()
                n198 = node-c288(w329) -> ()
              }
              frame 6 {
                w391 = u8 0
                n199 = node-c288() -> (w397:T4)  [unwired: 1 in]
                n200 = while {
                  shift-right: [w447] -> _
                  shift-left: w399 -> [w453]
                  tunnel: w395 -> [w454]
                  tunnel: w386 -> [w451]
                  tunnel: w399 -> [w450]
                  stop <- w449 continue-if-true
                  n201 = Increment(x=w453) -> (x+1=w455:u32)
                  n202 = Equal?(x=w453, y=w454) -> (x = y?=w448:bool)
                  n203 = xnode ("Memory Read")("Address"=w453) -> ("Data"=w452:i16)  [unwired: 1 in, 1 out]
                  n204 = Select(t=w450, s=w448, f=w455) -> (s? t:f=w447:u32)
                  n205 = call "Loop Timer19"("Count(Ticks)"=w451) -> ()  [unwired: 1 out]
                  n206 = Less?(x=w447, y=u32 4) -> (x < y?=w445:bool)
                  n207 = local write "Frame Trigger"(w445) -> ()
                  n208 = local read "Start Waveforms"() -> (w449:bool)
                  n209 = xnode "FPGA I/O Node"("Connector0/AO5"=w452) -> ()  [unwired: 1 in, 1 out]
                }
                n210 = while {
                  shift-right: [w423] -> _
                  shift-left: FALSE -> [w424]
                  shift-right: [w417] -> _
                  shift-left: w391 -> [w419]
                  tunnel: w393 -> [w418]
                  shift-right: [w401] -> _
                  shift-left: w389 -> [w414]
                  tunnel: w392 -> [w413]
                  shift-right: [w407] -> _
                  shift-left: w391 -> [w410]
                  tunnel: w390 -> [w406]
                  tunnel: w389 -> [w403]
                  tunnel: w386 -> [w402]
                  stop <- w425 continue-if-true
                  n211 = local read "End Linear Ramp"() -> (w423:bool)
                  n212 = Increment(x=w419) -> (x+1=w422:u8)
                  n213 = Greater?(x=w423, y=w424) -> (0:w421:bool)
                  n214 = Select(t=w422, s=w421, f=w419) -> (s? t:f=w416:u8)
                  n215 = Add(x=w413, y=w414) -> (x+y=w415:i16)
                  n216 = Increment(x=w410) -> (x+1=w411:u8)
                  n217 = Equal?(x=w416, y=w418) -> (x = y?=w412:bool)
                  n218 = Select(t=u8 0, s=w412, f=w416) -> (s? t:f=w417:u8)
                  n219 = Select(t=w411, s=w412, f=w410) -> (s? t:f=w408:u8)
                  n220 = Select(t=w415, s=w412, f=w414) -> (s? t:f=w409:i16)
                  n221 = call "Loop Timer21"("Count(Ticks)"=w402) -> ()  [unwired: 1 out]
                  n222 = Equal?(x=w408, y=w406) -> (x = y?=w405:bool)
                  n223 = local read "Start Waveforms"() -> (w425:bool)
                  n224 = Select(t=w403, s=w405, f=w409) -> (s? t:f=w401:i16)
                  n225 = xnode "FPGA I/O Node"("Connector0/AO3"=w401) -> ()  [unwired: 1 in, 1 out]
                  n226 = Select(t=u8 0, s=w405, f=w408) -> (s? t:f=w407:u8)
                }
                n227 = timed-loop {
                  timing: w397 -> [_]
                  timing-out: [_] -> w396
                  tunnel: w386 -> [w437]
                  tunnel: [w437] -> w387
                  tunnel: w398 -> [w438]
                  i -> [w440]
                  stop <- w439 stop-if-true
                  n228 = Equal?(x=w438, y=w440) -> (x = y?=w439:bool)
                }
                n229 = while {
                  shift-right: [w428] -> _
                  shift-left: w399 -> [w434]
                  tunnel: w400 -> [w435]
                  tunnel: w387 -> [w432]
                  tunnel: w399 -> [w431]
                  tunnel: w388 -> [w427]
                  stop <- w430 continue-if-true
                  n230 = Increment(x=w434) -> (x+1=w436:u32)
                  n231 = Equal?(x=w434, y=w435) -> (x = y?=w429:bool)
                  n232 = xnode ("Memory Read")("Address"=w434) -> ("Data"=w433:i16)  [unwired: 1 in, 1 out]
                  n233 = Select(t=w431, s=w429, f=w436) -> (s? t:f=w428:u32)
                  n234 = Greater?(x=w427, y=w428) -> (0:→"End Linear Ramp":bool)
                  n235 = call "Loop Timer20"("Count(Ticks)"=w432) -> ()  [unwired: 1 out]
                  n236 = local read "Start Waveforms"() -> (w430:bool)
                  n237 = xnode "FPGA I/O Node"("Connector0/AO6"=w433) -> ()  [unwired: 1 in, 1 out]
                }
                n238 = node-c288(w396) -> ()
              }
              frame 7 {
                w465 = u8 0
                n239 = node-c288() -> (w470:T4)  [unwired: 1 in]
                n240 = while {
                  shift-right: [w518] -> _
                  shift-left: w471 -> [w524]
                  tunnel: w458 -> [w525]
                  tunnel: w459 -> [w522]
                  tunnel: w471 -> [w521]
                  stop <- w520 continue-if-true
                  n241 = Increment(x=w524) -> (x+1=w526:u32)
                  n242 = Equal?(x=w524, y=w525) -> (x = y?=w519:bool)
                  n243 = xnode ("Memory Read")("Address"=w524) -> ("Data"=w523:i16)  [unwired: 1 in, 1 out]
                  n244 = Select(t=w521, s=w519, f=w526) -> (s? t:f=w518:u32)
                  n245 = call "Loop Timer4"("Count(Ticks)"=w522) -> ()  [unwired: 1 out]
                  n246 = Less?(x=w518, y=u32 20) -> (x < y?=w516:bool)
                  n247 = xnode "FPGA I/O Node"("TRIG0"=w516) -> ()  [unwired: 1 in, 1 out]
                  n248 = local read "Start Waveforms"() -> (w520:bool)
                  n249 = xnode "FPGA I/O Node"("Connector0/AO1"=w523) -> ()  [unwired: 1 in, 1 out]
                }
                n250 = while {
                  shift-right: [w472] -> _
                  shift-left: FALSE -> [w495]
                  shift-right: [w489] -> _
                  shift-left: w465 -> [w491]
                  tunnel: w467 -> [w490]
                  shift-right: [w473] -> _
                  shift-left: w463 -> [w486]
                  tunnel: w466 -> [w485]
                  shift-right: [w479] -> _
                  shift-left: w465 -> [w482]
                  tunnel: w464 -> [w478]
                  tunnel: w463 -> [w475]
                  tunnel: w460 -> [w474]
                  stop <- w496 continue-if-true
                  n251 = local read "End Linear Ramp"() -> (w472:bool)
                  n252 = Increment(x=w491) -> (x+1=w494:u8)
                  n253 = Greater?(x=w472, y=w495) -> (0:w493:bool)
                  n254 = Select(t=w494, s=w493, f=w491) -> (s? t:f=w488:u8)
                  n255 = Add(x=w485, y=w486) -> (x+y=w487:i16)
                  n256 = Increment(x=w482) -> (x+1=w483:u8)
                  n257 = Equal?(x=w488, y=w490) -> (x = y?=w484:bool)
                  n258 = Select(t=u8 0, s=w484, f=w488) -> (s? t:f=w489:u8)
                  n259 = Select(t=w483, s=w484, f=w482) -> (s? t:f=w480:u8)
                  n260 = Select(t=w487, s=w484, f=w486) -> (s? t:f=w481:i16)
                  n261 = call "Loop Timer17"("Count(Ticks)"=w474) -> ()  [unwired: 1 out]
                  n262 = Equal?(x=w480, y=w478) -> (x = y?=w477:bool)
                  n263 = local read "Start Waveforms"() -> (w496:bool)
                  n264 = Select(t=w475, s=w477, f=w481) -> (s? t:f=w473:i16)
                  n265 = xnode "FPGA I/O Node"("Connector0/AO3"=w473) -> ()  [unwired: 1 in, 1 out]
                  n266 = Select(t=u8 0, s=w477, f=w480) -> (s? t:f=w479:u8)
                }
                n267 = timed-loop {
                  timing: w470 -> [_]
                  timing-out: [_] -> w469
                  tunnel: w460 -> [w508]
                  tunnel: [w508] -> w461
                  tunnel: w457 -> [w509]
                  i -> [w511]
                  stop <- w510 stop-if-true
                  n268 = Equal?(x=w509, y=w511) -> (x = y?=w510:bool)
                }
                n269 = while {
                  shift-right: [w499] -> _
                  shift-left: w471 -> [w505]
                  tunnel: w456 -> [w506]
                  tunnel: w461 -> [w503]
                  tunnel: w471 -> [w502]
                  tunnel: w462 -> [w498]
                  stop <- w501 continue-if-true
                  n270 = Increment(x=w505) -> (x+1=w507:u32)
                  n271 = Equal?(x=w505, y=w506) -> (x = y?=w500:bool)
                  n272 = xnode ("Memory Read")("Address"=w505) -> ("Data"=w504:i16)  [unwired: 1 in, 1 out]
                  n273 = Select(t=w502, s=w500, f=w507) -> (s? t:f=w499:u32)
                  n274 = Greater?(x=w498, y=w499) -> (0:w497:bool)
                  n275 = local write "End Linear Ramp"(w497) -> ()
                  n276 = call "Loop Timer15"("Count(Ticks)"=w503) -> ()  [unwired: 1 out]
                  n277 = local read "Start Waveforms"() -> (w501:bool)
                  n278 = xnode "FPGA I/O Node"("Connector0/AO2"=w504) -> ()  [unwired: 1 in, 1 out]
                }
                n279 = node-c288(w469) -> ()
              }
            }
            n280 = Index Array(array="Accums Per Line", index #1=0 ("index"), index #2=1 ("index"), index #3=2 ("index"), index #4=3 ("index")) -> (element #1=w87:u32, element #2=w86:u32, element #3=w85:u32, element #4=w84:u32)
            n281 = Compound Arithmetic op=ADD(w87, w86, w85, w84) -> (w94:u32)
            n282 = case shown="3" w76 {
              frame 0, Default {
              }
              frame 3 {
                n283 = while {
                  stop <- w109 continue-if-true
                  n284 = local read "Start Waveforms"() -> (w109:bool)
                  n285 = xnode "FPGA I/O Node"("Connector0/AO1"="X Piezo Axis", "Connector0/AO2"="Y Piezo Axis", "Connector0/AO3"="Z Piezo Axis") -> ()  [unwired: 3 in, 3 out]
                }
              }
            }
            n286 = node-c288() -> (w97:T4)  [unwired: 1 in]
            n287 = Multiply(x="Number of Lines", y=w94) -> (x*y=w95:u32)
            n288 = timed-loop {
              timing: w97 -> [_]
              timing-out: [_] -> w96
              shift-right: [w129] -> _
              shift-left: w83 -> [w128]
              shift-right: [w126] -> _
              shift-left: _ -> [w119]
              shift-right: [w127] -> _
              shift-left: _ -> [w125]
              shift-right: [w111] -> _
              shift-left: u32 0 -> [w116]
              shift-right: [w121] -> _
              shift-left: w83 -> [w118]
              tunnel: w95 -> [w115]
              stop <- "Stop Sync Signal" continue-if-true
              n289 = Increment(x=w116) -> (x+1=w120:u32)
              n290 = Equal?(x=w116, y=w115) -> (x = y?=w113:bool)
              n291 = And(x=w119, y=w118) -> (x .and. y?=w124:bool)
              n292 = And(x=w118, y=w119) -> (x .and. y?=w117:bool)
              n293 = local read "Frame Trigger"() -> (w123:bool)
              n294 = case shown="True" w125 {
                tunnel: w124 -> [_ w130]
                frame False {
                }
                frame True {
                  n295 = xnode "FPGA I/O Node"("TRIG1"=w130) -> ()  [unwired: 1 in, 1 out]
                  "Laser Blank Trigger" <- w130
                }
              }
              n296 = Select(t=w120, s=w117, f=w116) -> (s? t:f=w114:u32)
              n297 = Exclusive Or(1:w113, 2:w123) -> (0:w122:bool)
              n298 = xnode "FPGA I/O Node"() -> ("Connector1/DIO0"=w129:bool)  [unwired: 1 in, 1 out]
              n299 = Select(t=w123, s=w122, f=w118) -> (s? t:f=w121:bool)
              n300 = Select(t=u32 0, s=w113, f=w114) -> (s? t:f=w111:u32)
              n301 = Not Equal?(x=w129, y=w128) -> (x != y?=w127:bool)
              n302 = Greater?(x=w129, y=w128) -> (0:w126:bool)
            }
            n303 = node-c288(w96) -> ()
          }
        }
      }
    }
  }
  n304 = local read "Accums Per Line"() -> (w1:u32[])
  n305 = while {
    shift-right: [w573] -> _
    shift-left: u8 0 -> [w550]
    shift-right: [w574] -> _
    shift-left: w2 -> [w578]
    shift-right: [w572] -> _
    shift-left: u8 0 -> [w575]
    tunnel: "Sequences" -> [w571]
    shift-right: [w565] -> _
    shift-left: u32 0 -> [w566]
    tunnel: w1 -> [w552]
    shift-right: [w545] -> _
    shift-left: w2 -> [w544]
    stop <- FALSE stop-if-true
    n306 = local read "Laser Blank Trigger"() -> (w545:bool)
    n307 = To Long Integer(number=w550) -> (32bit integer=w549:i32)
    n308 = Add(x="Laser Delay (Ticks)", y="Laser On Time (Ticks)") -> (x+y=w528:u8)
    n309 = Index Array(array=w552, index=w549) -> (element=w551:u32)
    n310 = Increment(x=w566) -> (x+1=w567:u32)
    n311 = Equal?(x=w566, y=w551) -> (x = y?=w563:bool)
    n312 = Equal?(x=w575, y=w528) -> (x = y?=w564:bool)
    n313 = Greater?(x=w545, y=w544) -> (0:w543:bool)
    n314 = Select(t=w567, s=w564, f=w566) -> (s? t:f=w568:u32)
    n315 = Increment(x=w550) -> (x+1=w583:u8)
    n316 = Equal?(x=w550, y=w571) -> (x = y?=w580:bool)
    n317 = Exclusive Or(1:w564, 2:w543) -> (0:w579:bool)
    n318 = Select(t=u32 0, s=w563, f=w568) -> (s? t:f=w565:u32)
    n319 = Select(t=w583, s=w563, f=w550) -> (s? t:f=w582:u8)
    n320 = Increment(x=w575) -> (x+1=w577:u8)
    n321 = Select(t=w543, s=w579, f=w578) -> (s? t:f=w574:bool)
    n322 = Split Number(x="Laser States") -> (hi(x)=w560:u16, lo(x)=w561:u16)
    n323 = Select(t=u8 0, s=w580, f=w582) -> (s? t:f=w573:u8)
    n324 = Select(t=w577, s=w574, f=u8 0) -> (s? t:f=w572:u8)
    n325 = Split Number(x=w560) -> (hi(x)=w559:u8, lo(x)=w558:u8)
    n326 = Split Number(x=w561) -> (hi(x)=w557:u8, lo(x)=w556:u8)
    n327 = Greater?(x=w572, y="Laser Delay (Ticks)") -> (0:w547:bool)
    n328 = call "Loop Timer22"("Count(Ticks)"=u16 80) -> ()  [unwired: 1 out]
    n329 = case shown="0, Default" w573 {
      tunnel: w559 -> [w584 _ _ _]
      tunnel: w558 -> [_ w585 _ _]
      tunnel: w557 -> [_ _ w586 _]
      tunnel: w556 -> [_ _ _ w587]
      tunnel: [w584 w585 w586 w587] -> w555
      frame 0, Default {
      }
      frame 1 {
      }
      frame 2 {
      }
      frame 3 {
      }
    }
    n330 = Or(x="Blanking Off/Manual", y=w547) -> (x .or. y?=w548:bool)
    n331 = Select(t=w555, s=w548, f=u8 0) -> (s? t:f=w540:u8)
    n332 = Number To Boolean Array(number=w540) -> (Boolean array=w542:bool[])
    n333 = Index Array(array=w542, index #1=0 ("index"), index #2=1 ("index"), index #3=2 ("index"), index #4=3 ("index")) -> (element #1=w532:bool, element #2=w531:bool, element #3=w533:bool, element #4=w530:bool)
    n334 = Select(t="590 Analog Voltage (I16)", s=w533, f=i16 0) -> (s? t:f=w538:i16)
    n335 = xnode "FPGA I/O Node"("Connector0/DIO0"=w532, "Connector1/DIO8"=w531, "Connector1/DIO9"=w530) -> ()  [unwired: 3 in, 3 out]
    n336 = xnode "FPGA I/O Node"("Connector0/AO0"=w538) -> ()  [unwired: 1 in, 1 out]
  }
